vi "Read.vi"(8 "error in (no error)":errorcluster, 11 "Save as ini in":refnum<class "Save as ini.lvclass">) -> (0 "error out":errorcluster, 1 "Data(UTF8)":string[][](array[string]), 2 "Data":string[][](array[string]), 3 "Save as ini out":refnum<class "Save as ini.lvclass">)   [LabVIEW 2020, in "Save as ini.lvclass"]
uses:
  Save as ini.lvclass
  Saving OO.lvclass
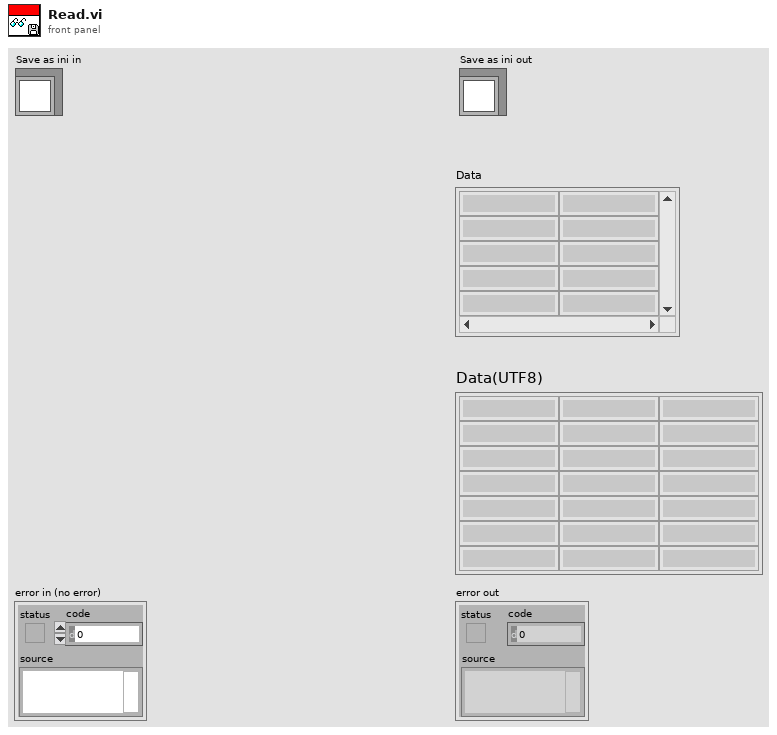
[diagram p1: front panel]
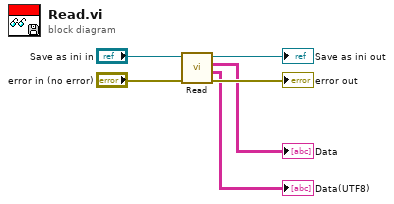
[diagram p0: block diagram]
diagram:
  n1 = call-parent "Read.vi"("error in (no error)"="error in (no error)", "Saving OO in"="Save as ini in") -> ("error out"=→"error out":errorcluster, "Data(UTF8)"=→"Data(UTF8)":string[][], "Data(Text)"=→"Data":string[][], "Saving OO out"=→"Save as ini out":refnum<class "Save as ini.lvclass">)  [unwired: 6 in]
